vi "Run All.vi"(8 "Error In":errorcluster) -> (0 "Error Out":errorcluster)   [LabVIEW 2017, in "Tests.lvlib" / "To Msgpack.lvlib"]
uses:
  To Msgpack.lvlib
  <vilib>/addons/_JKI Toolkits/Caraya/classes/Test/Test.lvclass
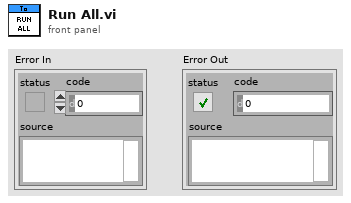
[diagram p1: front panel]
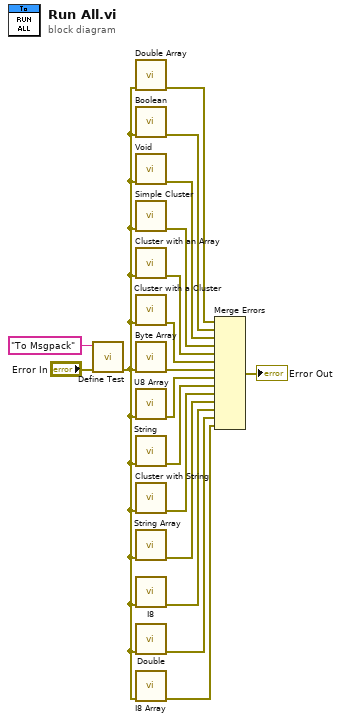
[diagram p0: block diagram]
diagram:
  n1 = call <vilib>:"Define Test.vi"("error in (no error)"="Error In", "Label (VI Title)"="To Msgpack") -> ("error out"=w2:errorcluster)  [unwired: 9 in]
  n2 = call "Double Array.vi"("Error In"=w2) -> ("Error Out"=w16:errorcluster)  [unwired: 10 in]
  n3 = call "Boolean.vi"("Error In"=w2) -> ("Error Out"=w14:errorcluster)  [unwired: 10 in]
  n4 = call "Void.vi"("Error In"=w2) -> ("Error Out"=w13:errorcluster)  [unwired: 10 in]
  n5 = call "Simple Cluster.vi"("Error In"=w2) -> ("Error Out"=w12:errorcluster)  [unwired: 10 in]
  n6 = call "Cluster with an Array.vi"("Error In"=w2) -> ("Error Out"=w11:errorcluster)  [unwired: 10 in]
  n7 = call "Cluster with a Cluster.vi"("Error In"=w2) -> ("Error Out"=w10:errorcluster)  [unwired: 10 in]
  n8 = call "Byte Array.vi"("Error In"=w2) -> ("Error Out"=w9:errorcluster)  [unwired: 10 in]
  n9 = call "U8 Array.vi"("Error In"=w2) -> ("Error Out"=w8:errorcluster)  [unwired: 10 in]
  n10 = call "String.vi"("Error In"=w2) -> ("Error Out"=w7:errorcluster)  [unwired: 10 in]
  n11 = call "Cluster with String.vi"("Error In"=w2) -> ("Error Out"=w6:errorcluster)  [unwired: 10 in]
  n12 = call "String Array.vi"("Error In"=w2) -> ("Error Out"=w5:errorcluster)  [unwired: 10 in]
  n13 = call "I8.vi"("Error In"=w2) -> ("Error Out"=w4:errorcluster)  [unwired: 10 in]
  n14 = call "Double.vi"("Error In"=w2) -> ("Error Out"=w3:errorcluster)  [unwired: 10 in]
  n15 = call "I8 Array.vi"("Error In"=w2) -> ("Error Out"=w1:errorcluster)  [unwired: 10 in]
  n16 = Merge Errors(w16, w14, w13, w12, w11, w10, w9, w8, w7, w6, w5, w4, w3, w1) -> (→"Error Out":errorcluster)
